vi "SPC_get_parameters.vi"(8 "Error In":errorcluster, 10 "Module No":i16 min=0 max=7 step=1, 11 "DLL Path":path) -> (0 "Error Out":errorcluster, 2 "Module No":i16, 3 "DLL Path":path, 5 "SPCdata":T1={"base_adr"=896, "init"=0, "cfd_limit_low"=5.0, "cfd_limit_high"=80.0, "cfd_zc_level"=0.0, "cfd_holdoff"=5.0, "sync_zc_level"=0.0, "sync_holdoff"=4.0, "sync_threshold"=-20.0, "tac_range"=50.0, "sync_freq_div"=1, "tac_gain"=1, "tac_offset"=0.0, "tac_limit_low"=10.0, "tac_limit_high"=80.0, "adc_resolution"=10, "ext_latch_delay"=0, "collect_time"=0.01, "display_time"=1.0, "repeat_time"=10.0001, "stop_on_time"=1, "stop_on_ovfl"=1, "dither_range"=0, "count_incr"=1, "mem_bank"=0, "dead_time_comp"=1, "scan_control"=61440, "routing_mode"=0, "tac_enable_hold"=10.0, "pci_card_no"=-1, "mode"=0, "scan_size_x"=1, "scan_size_y"=1, "scan_rout_x"=1, "scan_rout_y"=1, "scan_flyback"=0, "scan_borders"=0, "scan_polarity"=0, "pixel_clock"=0, "line_compression"=1, "trigger"=0, "pixel_time"=5e-08, "ext_pixclk_div"=1, "rate_count_time"=1.0, "macro_time_clk"=0, "add_select"=0, "test_eep"=0, "adc_zoom"=0, "img_size_x"=1, "img_size_y"=1, "img_rout_x"=1, "img_rout_y"=1, "xy_gain"=1, "master_clock"=0, "adc_sample_delay"=0, "detector_type"=1, "chan_enable"=4191231, "chan_slope"=0, "chan_spec_no"=34835, "tdc_control"=0, "tdc_offset1"=0.0, "tdc_offset2"=0.0, "tdc_offset3"=0.0, "tdc_offset4"=0.0, "tdc_offset5"=0.0, "tdc_offset6"=0.0, "cfd_th5_tdc"=0.0, "cfd_th6_tdc"=0.0, "cfd_zc5_tdc"=0.0, "cfd_zc6_tdc"=0.0, "future_reserve1"=0, "future_reserve2"=0, "future_reserve3"=0, "future_reserve4"=0})   [LabVIEW 2023]
doc: "After calling the SPC_init function (see above) the measurement parameters from the \ninitialisation file are present in the module and in the internal data structures of the DLLs. To \ngive the user access to the parameters, the function SPC_get_parameters is provided. This \nfunction transfers the parameter values from the internal DLL structures of the module \n‘mod_no’ into a structure of the type SPCdata (see spcm_def.h) which has to be defined by the \nuser. The parameter values in this structure are described in spcm_def.h\n\ninfo@becker-hickl.com"
uses:
  SPC_Controls/SPCdata.ctl
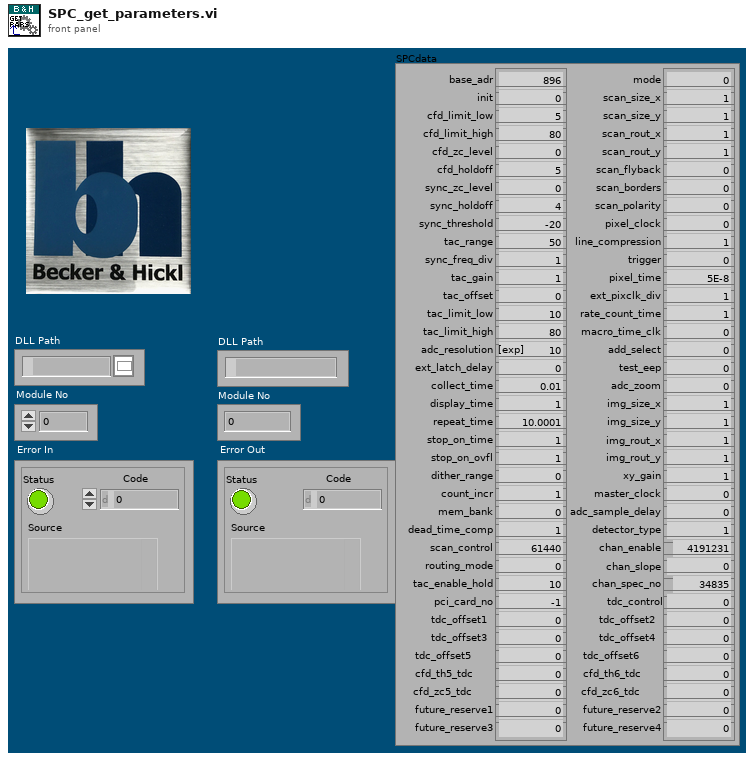
[diagram p1: front panel]
types:
  T1 = typedef "SPCdata.ctl" = cluster{"base_adr":u16, "init":i16, "cfd_limit_low":sgl, "cfd_limit_high":sgl, "cfd_zc_level":sgl, "cfd_holdoff":sgl, "sync_zc_level":sgl, "sync_holdoff":sgl, "sync_threshold":sgl, "tac_range":sgl, "sync_freq_div":i16, "tac_gain":i16, "tac_offset":sgl, "tac_limit_low":sgl, "tac_limit_high":sgl, "adc_resolution":i16, "ext_latch_delay":i16, "collect_time":sgl, "display_time":sgl, "repeat_time":sgl, "stop_on_time":i16, "stop_on_ovfl":i16, "dither_range":i16, "count_incr":i16, "mem_bank":i16, "dead_time_comp":i16, "scan_control":u16, "routing_mode":u16, "tac_enable_hold":sgl, "pci_card_no":i16, "mode":u16, "scan_size_x":u32, "scan_size_y":u32, "scan_rout_x":u32, "scan_rout_y":u32, "scan_flyback":u32, "scan_borders":u32, "scan_polarity":u16, "pixel_clock":u16, "line_compression":u16, "trigger":u16, "pixel_time":sgl, "ext_pixclk_div":u32, "rate_count_time":sgl, "macro_time_clk":i16, "add_select":i16, "test_eep":i16, "adc_zoom":i16, "img_size_x":u32, "img_size_y":u32, "img_rout_x":u32, "img_rout_y":u32, "xy_gain":i16, "master_clock":i16, "adc_sample_delay":i16, "detector_type":i16, "chan_enable":u32, "chan_slope":u32, "chan_spec_no":u32, "tdc_control":u32, "tdc_offset1":sgl, "tdc_offset2":sgl, "tdc_offset3":sgl, "tdc_offset4":sgl, "tdc_offset5":sgl, "tdc_offset6":sgl, "cfd_th5_tdc":sgl, "cfd_th6_tdc":sgl, "cfd_zc5_tdc":sgl, "cfd_zc6_tdc":sgl, "future_reserve1":u64, "future_reserve2":u64, "future_reserve3":u64, "future_reserve4":u64}
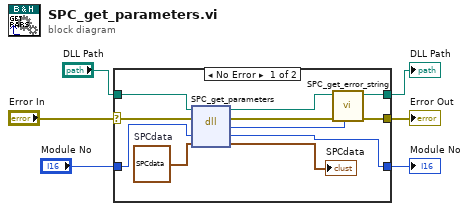
[diagram p0: block diagram]
diagram:
  n1 = case shown="No Error" "Error In" {
    selector: "Error In" -> [w15 w19]
    tunnel: "DLL Path" -> [w17 w20]
    tunnel: [w10 w20] -> w5
    tunnel: [w7 w19] -> w3
    tunnel: [w13 w18] -> w2
    tunnel: "Module No" -> [w12 w18]
    frame No Error {
      w14 = T1 {"base_adr"=896, "init"=0, "cfd_limit_low"=5.0, "cfd_limit_high"=80.0, "cfd_zc_level"=0.0, "cfd_holdoff"=5.0, "sync_zc_level"=0.0, "sync_holdoff"=4.0, "sync_threshold"=-20.0, "tac_range"=50.0, "sync_freq_div"=1, "tac_gain"=1, "tac_offset"=0.0, "tac_limit_low"=10.0, "tac_limit_high"=80.0, "adc_resolution"=10, "ext_latch_delay"=0, "collect_time"=0.01, "display_time"=1.0, "repeat_time"=10.0001, "stop_on_time"=1, "stop_on_ovfl"=1, "dither_range"=0, "count_incr"=1, "mem_bank"=0, "dead_time_comp"=1, "scan_control"=61440, "routing_mode"=0, "tac_enable_hold"=10.0, "pci_card_no"=-1, "mode"=0, "scan_size_x"=1, "scan_size_y"=1, "scan_rout_x"=1, "scan_rout_y"=1, "scan_flyback"=0, "scan_borders"=0, "scan_polarity"=0, "pixel_clock"=0, "line_compression"=1, "trigger"=0, "pixel_time"=5e-08, "ext_pixclk_div"=1, "rate_count_time"=1.0, "macro_time_clk"=0, "add_select"=0, "test_eep"=0, "adc_zoom"=0, "img_size_x"=1, "img_size_y"=1, "img_rout_x"=1, "img_rout_y"=1, "xy_gain"=1, "master_clock"=0, "adc_sample_delay"=0, "detector_type"=1, "chan_enable"=4191231, "chan_slope"=0, "chan_spec_no"=34835, "tdc_control"=0, "tdc_offset1"=0.0, "tdc_offset2"=0.0, "tdc_offset3"=0.0, "tdc_offset4"=0.0, "tdc_offset5"=0.0, "tdc_offset6"=0.0, "cfd_th5_tdc"=0.0, "cfd_th6_tdc"=0.0, "cfd_zc5_tdc"=0.0, "cfd_zc6_tdc"=0.0, "future_reserve1"=0, "future_reserve2"=0, "future_reserve3"=0, "future_reserve4"=0}  # SPCdata
      n2 = dll-call lib="D:/spcm/lib/lab_view/lv10.0/spcm32.dll" fn="SPC_get_parameters"(path in=w17, error in=w15, "mod_no"=w12, "data"=w14) -> (path out=w16:path, error out=w8:errorcluster, "return type"=w9:i16, "mod_no"=w13:i16, "data"=→"SPCdata":T1)  [unwired: 1 in]
      n3 = call "SPC_get_error_string.vi"("ErrorID"=w9, "Error In"=w8, "DLL Path"=w16) -> ("Error Out"=w7:errorcluster, "DLL Path"=w10:path)  [unwired: 6 in, 1 out]
    }
    frame Error {
    }
  }
  "DLL Path" <- w5
  "Error Out" <- w3
  "Module No" <- w2
